vi "Periodic Tasks.vi"(8 "error in":errorcluster) -> ()   [LabVIEW 2018]
doc: "This VI runs in parallel to other tasks. It can contain as many user-defined periodic loops as you need. These can carry out PID or other sorts of timed response."
uses:
  <vilib>/Rock Robotics/WPI/Utilities/WPI_GetSetVariantRefNum.vi
  <vilib>/Rock Robotics/WPI/Ultrasonic/WPI_SonarSRF04DigitalRefNum Registry Get.vi
  <vilib>/Rock Robotics/Network Tables/NT Read Boolean.vi
  <vilib>/Rock Robotics/Network Tables/NT Write Boolean.vi
  <vilib>/Rock Robotics/WPI/Ultrasonic/WPI_SonarSRF04DigitalGetRange.vi
  <vilib>/Rock Robotics/Network Tables/NT Write Number.vi
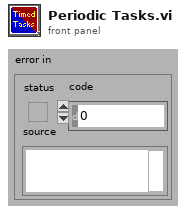
[diagram p1: front panel]
types:
  T1 = typedef "WPI_EncoderDevRef.ctl" = cluster{"DevStatus":errorcluster, "EncoderIndex":T2, "CounterIndex":T3, "DistancePerCount":dbl, "Decoding Type":T4}
  T2 = typedef "FPGA_EncoderIdx.ctl" = enum8{"Enc 0", "Enc 1", "Enc 2", "Enc 3", "Enc 4", "Enc 5", "Enc 6", "Enc 7", "Invalid"}
  T3 = typedef "FPGA_CounterCtrSystemIndex.ctl" = enum8{"Ctr 0", "Ctr 1", "Ctr 2", "Ctr 3", "Ctr 4", "Ctr 5", "Ctr 6", "Ctr 7", "Invalid"}
  T4 = typedef "WPI_EncoderType.ctl" = enum16{"1x", "2x", "4x"}
  T5 = typedef "WPI_JoystickDevRef.ctl" = cluster{"Device":T6}
  T6 = typedef "WPI_JoystickDeviceEnum.ctl" = enum16{"USB 0", "USB 1", "USB 2", "USB 3", "USB 4", "USB 5"}
  T7 = typedef "WPI_RobotDriveDevRef.ctl" = cluster{"DevStatus":errorcluster, "Motors[]":T8[], "Square Inputs":bool, "Max Output":dbl}
  T8 = typedef "WPI_MotorControlDeviceRef.ctl" = cluster{"DeviceStatus":errorcluster, "Type":T9, "PWM":cluster{"PWM Channel":T10, "DeadBand":T11}, "CAN":cluster{"Device Number":u8, "SetOutput VI Ref":variant, "GetOutput VI Ref":variant, "Enable VI Ref":variant, "Disable VI Ref":variant, "Data":variant}, "Invert":bool, "DIO PWM":cluster{"PWM \"Enable\" Channel":T10, "DIOChannel":T12, "PWM Rate":dbl}}
  T9 = typedef "WPI_MotorControlType.ctl" = enum16{"PWM", "CAN", "DIO PWM"}
  T10 = typedef "FPGA_DIOPWMChannel.ctl" = enum8{"PWM 0", "PWM 1", "PWM 2", "PWM 3", "PWM 4", "PWM 5", "PWM 6", "PWM 7", "PWM 8", "PWM 9", "PWM MXP 0", "PWM MXP 1", "PWM MXP 2", "PWM MXP 3", "PWM MXP 4", "PWM MXP 5", "PWM MXP 6", "PWM MXP 7", "PWM MXP 8", "PWM MXP 9", "Invalid"}
  T11 = typedef "WPI_PWMDeadband.ctl" = cluster{"Name":string, "maxPositivePwm":i32, "minPositivePwm":i32, "centerPwm":i32, "maxNegativePwm":i32, "minNegativePwm":i32, "angularRange":u16}
  T12 = typedef "FPGA_DIOChannel.ctl" = enum8{"DIO 0", "DIO 1", "DIO 2", "DIO 3", "DIO 4", "DIO 5", "DIO 6", "DIO 7", "DIO 8", "DIO 9", "DIO MXP 0", "DIO MXP 1", "DIO MXP 2", "DIO MXP 3", "DIO MXP 4", "DIO MXP 5", "DIO MXP 6", "DIO MXP 7", "DIO MXP 8", "DIO MXP 9", "DIO MXP 10", "DIO MXP 11", "DIO MXP 12", "DIO MXP 13", "DIO MXP 14", "DIO MXP 15", "SPI Port CS1", "SPI Port CS2", "SPI Port CS3", "SPI Port MISO", "SPI Port MOSI", "Invalid"}
  T13 = typedef "WPI_UltrasonicDeviceRef.ctl" = cluster{"DevStatus":errorcluster, "Ping Channel":T12, "Echo Channel":T12, "CntIndex":T3}
  T14 = typedef "WPI_SwitchDevRef.ctl" = cluster{"DevStatus":errorcluster, "DIO Channel":T12, "CntIndex":T3, "Normally Closed":bool}
  T15 = cluster{"JoystickDevRef":T5, "RobotDriveDevRef":T7}
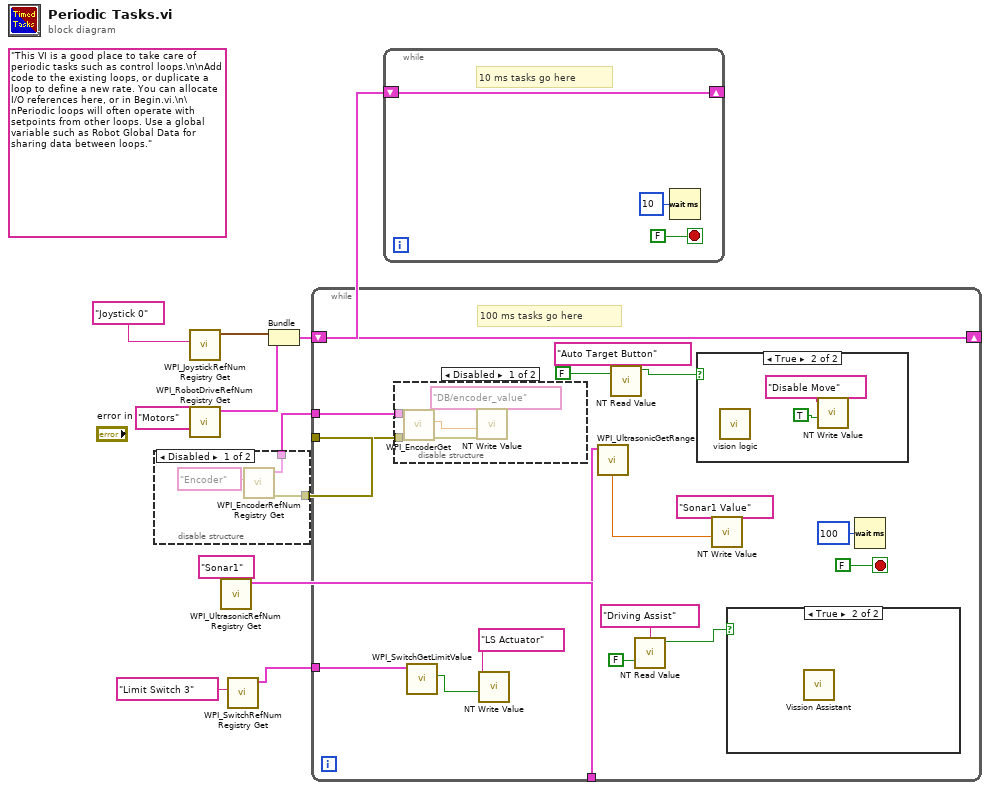
[diagram p0: block diagram]
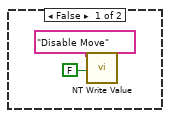
[diagram p4: hidden frame]
diagram:
  (unwired) "This VI is a good place to take care of periodic tasks such as control loops.\n\nAdd code to the existing loops, or duplicate a loop to define a new rate. You can allocate I/O references here, or in Begin.vi.\n\nPeriodic loops will often operate with setpoints from other loops. Use a global variable such as Robot Global Data for sharing data between loops."
  n1 = disable-structure shown="Disabled" {
    disable-tunnel: [w13 _] -> w6
    disable-tunnel: [w12 _] -> w5
    frame Disabled {
      n2 = call <vilib>:"WPI_EncoderRefNum Registry Get.vi"("refnum name"="Encoder") -> ("error out"=w12:errorcluster, "EncoderDevRef"=w13:T1)  [unwired: 9 in]
    }
    frame Enabled {
    }
  }
  n3 = call <vilib>:"WPI_JoystickRefNum Registry Get.vi"("refnum name"="Joystick 0") -> ("JoystickDevRef"=w9:T5)  [unwired: 1 in, 9 out]
  n4 = call <vilib>:"WPI_RobotDriveRefNum Registry Get.vi"("refnum name"="Motors") -> ("RobotDriveDevRef"=w8:T7)  [unwired: 1 in, 9 out]
  n5 = call-poly <vilib>:"WPI_UltrasonicRefNum Registry Get.vi"("refnum name"="Sonar1") -> ("SonarSRF04DevRef"=w3:T13)  [unwired: 9 in, 1 out]
  n6 = call <vilib>:"WPI_SwitchRefNum Registry Get.vi"("refnum name"="Limit Switch 3") -> ("SwitchDevRef"=w1:T14)  [unwired: 9 in, 1 out]
  n7 = Bundle("JoystickDevRef"=w9, "RobotDriveDevRef"=w8) -> (w7:T15)  [unwired: 1 out]
  n8 = while {
    shift-right: [w29] -> _
    shift-left: w7 -> [w29]
    tunnel: w6 -> [w28]
    tunnel: w5 -> [w27]
    tunnel: w3 -> [w26]
    tunnel: w1 -> [w20]
    stop <- FALSE stop-if-true
    # "100 ms tasks go here"
    n9 = disable-structure shown="Disabled" {
      disable-tunnel: w28 -> [w40 _]
      disable-tunnel: w27 -> [w36 _]
      frame Disabled {
        n10 = call <vilib>:"WPI_EncoderGet.vi"("error in (no error)"=w36, "EncoderDevRef"=w40) -> ("error out"=w37:errorcluster, "Distance"=w39:dbl)  [unwired: 4 in, 4 out]
        n11 = call-poly <vilib>:"NT Write Value.vi"("error in"=w37, "Numeric"=w39, "Name"="DB/encoder_value") -> ()  [unwired: 8 in, 1 out]
      }
      frame Enabled {
      }
    }
    n12 = call <vilib>:"WPI_SwitchGetLimitValue.vi"("SwitchDevRef"=w20) -> ("Switch Pressed"=w19:bool)  [unwired: 8 in, 2 out]
    n13 = call-poly <vilib>:"NT Write Value.vi"("Boolean"=w19, "Name"="LS Actuator") -> ()  [unwired: 9 in, 1 out]
    n14 = call-poly <vilib>:"WPI_UltrasonicGetRange.vi"("SonarSRF04DevRef"=w26) -> ("Distance"=w25:dbl)  [unwired: 8 in, 2 out]
    n15 = call-poly <vilib>:"NT Read Value.vi"("Default Value"=FALSE, "Name"="Auto Target Button") -> ("Boolean"=w22:bool)  [unwired: 8 in, 1 out]
    n16 = call-poly <vilib>:"NT Read Value.vi"("Default Value"=FALSE, "Name"="Driving Assist") -> ("Boolean"=w15:bool)  [unwired: 8 in, 1 out]
    n17 = case shown="True" w22 {
      frame False {
        n18 = call-poly <vilib>:"NT Write Value.vi"("Boolean"=FALSE, "Name"="Disable Move") -> ()  [unwired: 9 in, 1 out]
      }
      frame True {
        n19 = call "vision logic.vi"() -> ()  [unwired: 16 in]
        n20 = call-poly <vilib>:"NT Write Value.vi"("Boolean"=TRUE, "Name"="Disable Move") -> ()  [unwired: 9 in, 1 out]
      }
    }
    n21 = call-poly <vilib>:"NT Write Value.vi"("Numeric"=w25, "Name"="Sonar1 Value") -> ()  [unwired: 9 in, 1 out]
    n22 = case shown="True" w15 {
      frame False {
      }
      frame True {
        n23 = call "Vission Assistant.vi"() -> ()  [unwired: 12 in]
      }
    }
    n24 = Wait (ms)(milliseconds to wait=u32 100) -> ()  [unwired: 1 out]
  }
  n25 = while {
    shift-right: [w41] -> _
    shift-left: w7 -> [w41]
    stop <- FALSE stop-if-true
    # "10 ms tasks go here"
    n26 = Wait (ms)(milliseconds to wait=u32 10) -> ()  [unwired: 1 out]
  }
